vi "initialize.vi"(0 "HGF_ThreadPool":refnum<class "HGF_ThreadPool.lvclass">, 3 "initializationData":variant, 5 "error in (no error)":errorcluster, 7 "binaryString":string, 8 "I8 Array":i8[](array[numeric]), 9 "prependSize? (T)":bool, 11 "byteOrder (0:big-endian, network order)":T1(ring)) -> (14 "dup HGF_ThreadPool":refnum<class "HGF_ThreadPool.lvclass">, 17 "found?":bool, 19 "error out":errorcluster)   [LabVIEW 2014, in "HGF_BaseClasses.lvlib" / "HGF_ThreadPool.lvclass"]
doc: "This is a dynamic dispatch VI to be implemented by child classes to initialize their attributes.\n\n<B>Recommendation:</B> Use Variant for initialization data."
uses:
  HGF_ThreadPool.lvclass
  HGF_Base/HGF_Base.lvclass
  HGF_ThreadWorker/HGF_ThreadWorker.lvclass
  HGF_ThreadTask/HGF_ThreadTask.lvclass
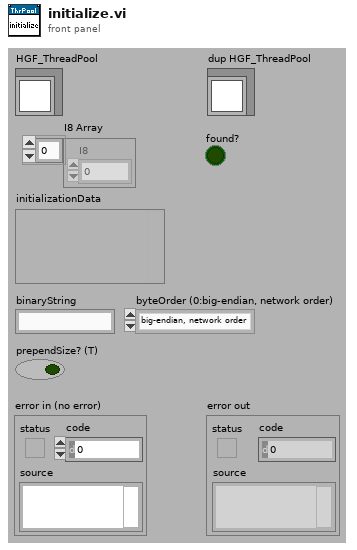
[diagram p1: front panel]
types:
  T1 = enum16{"big-endian, network order", "native, host order", "little-endian"}
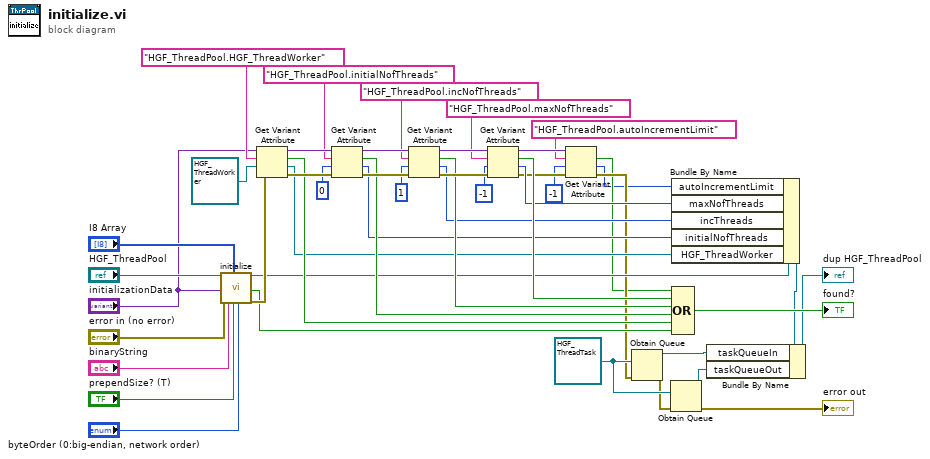
[diagram p0: block diagram]
diagram:
  w17 = refnum<class "HGF_ThreadTask.lvclass"> refnum ("HGF_BaseClasses.lvlib:HGF_ThreadTask.lvclass")
  n1 = call-parent "initialize.vi"("HGF_Base"="HGF_ThreadPool", "initializationData"="initializationData", "error in (no error)"="error in (no error)", "binaryString"="binaryString", "I8 Array"="I8 Array", "prependSize? (T)"="prependSize? (T)", "byteOrder (0:big-endian, network order)"="byteOrder (0:big-endian, network order)") -> ("dup HGF_Base"=w22:refnum<class "HGF_ThreadPool.lvclass">, "found?"=w34:bool, "error out"=w40:errorcluster)  [unwired: 1 in, 9 out]
  n2 = Get Variant Attribute(Variant="initializationData", name="HGF_ThreadPool.HGF_ThreadWorker", default value (empty Variant)=refnum<class "HGF_ThreadWorker.lvclass"> refnum ("HGF_ThreadWorker"), error in=w40) -> (duplicate Variant=w39:variant, found=w29:bool, value=w21:refnum<class "HGF_ThreadWorker.lvclass">, error out=w32:errorcluster)
  n3 = Get Variant Attribute(Variant=w39, name="HGF_ThreadPool.initialNofThreads", default value (empty Variant)=0 ("initialNofThreads"), error in=w32) -> (duplicate Variant=w38:variant, found=w28:bool, value=w20:i32, error out=w31:errorcluster)
  n4 = Get Variant Attribute(Variant=w38, name="HGF_ThreadPool.incNofThreads", default value (empty Variant)=1 ("incThreads"), error in=w31) -> (duplicate Variant=w37:variant, found=w27:bool, value=w19:i32, error out=w30:errorcluster)
  n5 = Get Variant Attribute(Variant=w37, name="HGF_ThreadPool.maxNofThreads", default value (empty Variant)=-1 ("maxNofThreads"), error in=w30) -> (duplicate Variant=w4:variant, found=w26:bool, value=w18:i32, error out=w10:errorcluster)
  n6 = Get Variant Attribute(Variant=w4, name="HGF_ThreadPool.autoIncrementLimit", default value (empty Variant)=-1 ("maxNofThreads")) -> (found=w3:bool, value=w2:i32)  [unwired: 1 in, 2 out]
  n7 = Obtain Queue(element data type=w17, error in (no error)=w10) -> (queue out=w14:refnum<queue>, error out=w16:errorcluster)  [unwired: 2 in, 2 out]
  n8 = Obtain Queue(element data type=w17, error in (no error)=w16) -> (queue out=w13:refnum<queue>, error out=→"error out":errorcluster)  [unwired: 2 in, 2 out]
  n9 = Bundle By Name(cluster=w22, "autoIncrementLimit"=w2, "maxNofThreads"=w18, "incThreads"=w19, "initialNofThreads"=w20, "HGF_ThreadWorker"=w21) -> (w11:refnum<class "HGF_ThreadPool.lvclass">)
  n10 = Compound Arithmetic op=OR(w3, w26, w27, w28, w29, w34) -> (→"found?":bool)
  n11 = Bundle By Name(cluster=w11, "taskQueueIn"=w14, "taskQueueOut"=w13) -> (→"dup HGF_ThreadPool":refnum<class "HGF_ThreadPool.lvclass">)
